vi "Set Aircraft Attitude.vi"(7 "Aircraft ID":u8, 8 "Error In":errorcluster, 11 "Aircraft Att Data In":T1) -> (0 "Error Out":errorcluster, 3 "Aircraft Att Data Out":T1)   [LabVIEW 2014]
uses:
  Controls/Aircraft Attitude Data.ctl
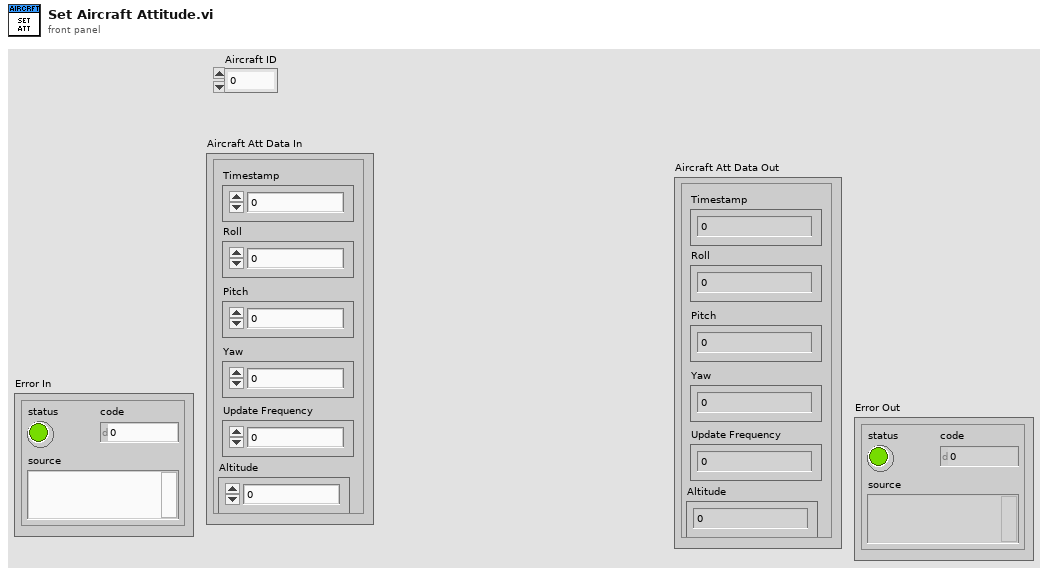
[diagram p1: front panel]
types:
  T1 = typedef "Aircraft Attitude Data.ctl" = cluster{"Roll":sgl, "Pitch":sgl, "Yaw":sgl, "Timestamp":u32, "Update Frequency":dbl, "Altitude":sgl}
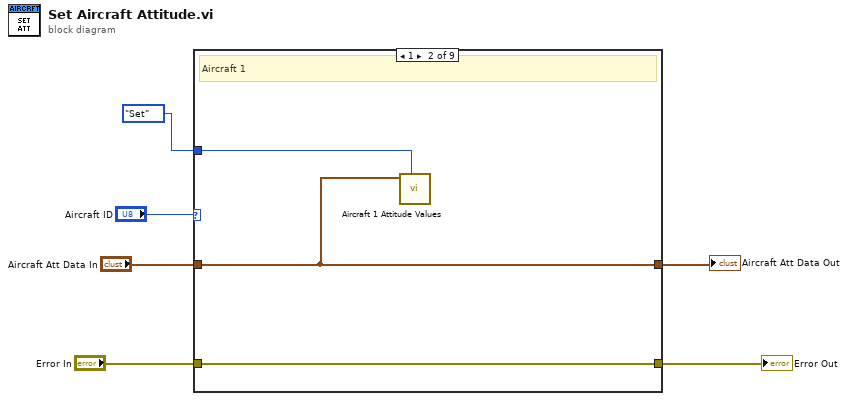
[diagram p0: block diagram]
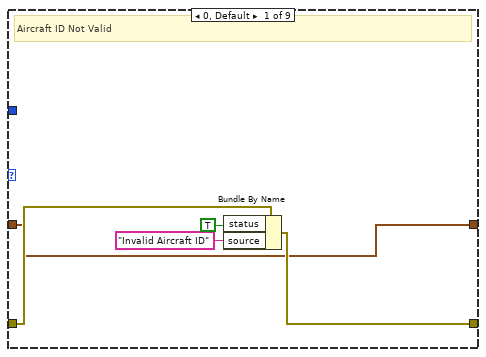
[diagram p2: hidden frame]
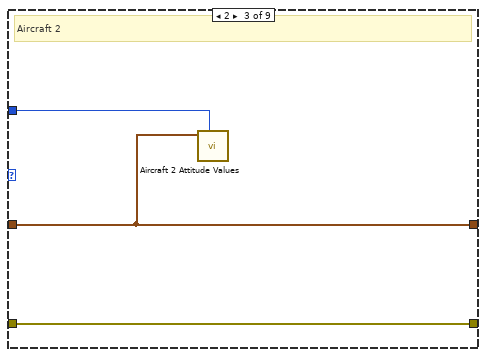
[diagram p3: hidden frame]
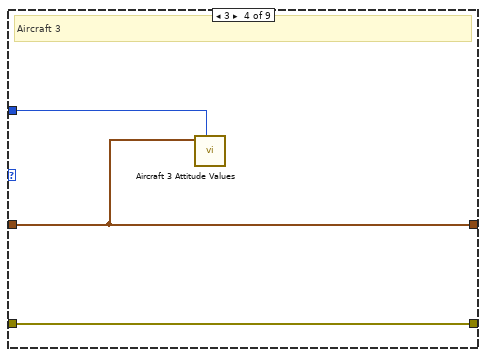
[diagram p4: hidden frame]
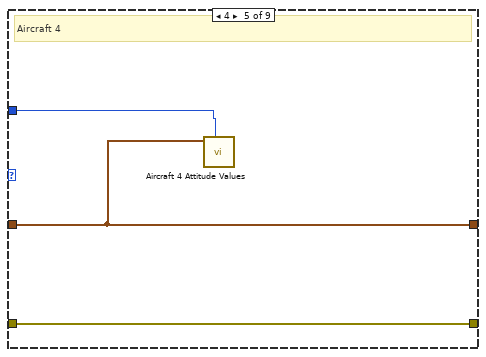
[diagram p5: hidden frame]
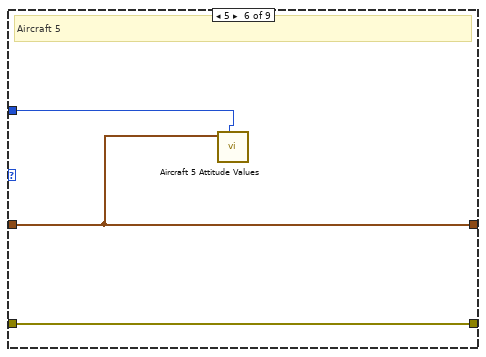
[diagram p6: hidden frame]
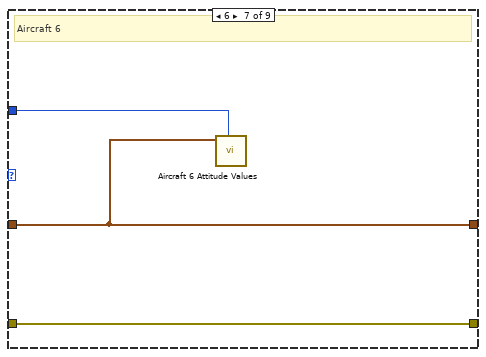
[diagram p7: hidden frame]
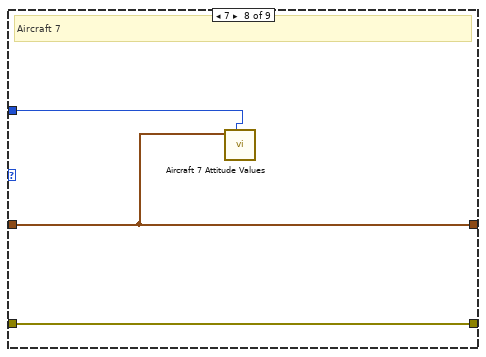
[diagram p8: hidden frame]
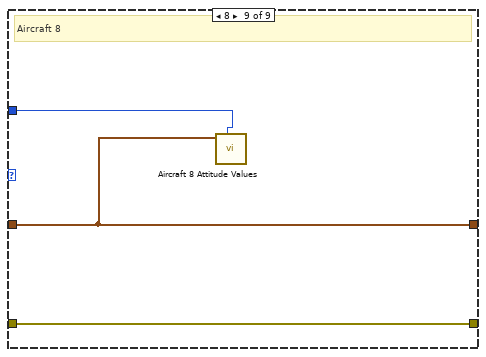
[diagram p9: hidden frame]
diagram:
  n1 = case shown="1" "Aircraft ID" {
    tunnel: [w10 w14 w17 w20 w23 w26 w29 w32 w35] -> w5
    tunnel: "Error In" -> [w11 w14 w17 w20 w23 w26 w29 w32 w35]
    tunnel: enum16{"Get", "Set"}."Set" ("Method") -> [_ w13 w16 w19 w22 w25 w28 w31 w34]
    tunnel: "Aircraft Att Data In" -> [w7 w12 w15 w18 w21 w24 w27 w30 w33]
    tunnel: [w7 w12 w15 w18 w21 w24 w27 w30 w33] -> w1
    frame 0, Default {
      # "Aircraft ID Not Valid"
      n2 = Bundle By Name(cluster=w11, "status"=TRUE, "source"="Invalid Aircraft ID") -> (w10:errorcluster)
    }
    frame 1 {
      # "Aircraft 1"
      n3 = call "Aircraft 1 Attitude Values .vi"("Method"=w13, "Aircraft Att Data"=w12) -> ()  [unwired: 9 in, 1 out]
    }
    frame 2 {
      # "Aircraft 2"
      n4 = call "Aircraft 2 Attitude Values .vi"("Method"=w16, "Aircraft Att Data"=w15) -> ()  [unwired: 9 in, 1 out]
    }
    frame 3 {
      # "Aircraft 3"
      n5 = call "Aircraft 3 Attitude Values .vi"("Method"=w19, "Aircraft Att Data"=w18) -> ()  [unwired: 9 in, 1 out]
    }
    frame 4 {
      # "Aircraft 4"
      n6 = call "Aircraft 4 Attitude Values .vi"("Method"=w22, "Aircraft Att Data"=w21) -> ()  [unwired: 9 in, 1 out]
    }
    frame 5 {
      # "Aircraft 5"
      n7 = call "Aircraft 5 Attitude Values .vi"("Method"=w25, "Aircraft Att Data"=w24) -> ()  [unwired: 9 in, 1 out]
    }
    frame 6 {
      # "Aircraft 6"
      n8 = call "Aircraft 6 Attitude Values .vi"("Method"=w28, "Aircraft Att Data"=w27) -> ()  [unwired: 9 in, 1 out]
    }
    frame 7 {
      # "Aircraft 7"
      n9 = call "Aircraft 7 Attitude Values .vi"("Method"=w31, "Aircraft Att Data"=w30) -> ()  [unwired: 9 in, 1 out]
    }
    frame 8 {
      # "Aircraft 8"
      n10 = call "Aircraft 8 Attitude Values .vi"("Method"=w34, "Aircraft Att Data"=w33) -> ()  [unwired: 9 in, 1 out]
    }
  }
  "Error Out" <- w5
  "Aircraft Att Data Out" <- w1
